vi "ProyectoInvernadero.vi"() -> ()   [LabVIEW 2020]
uses:
  <vilib>/Instr/_visa.llb/VISA Configure Serial Port (Instr).vi
  <vilib>/addons/Fuzzy Logic/FL Fuzzy Controller (SISO).vi
  <vilib>/addons/Fuzzy Logic/NI_Fuzzy_Logic_API.lvlib
panel:
  out "Error":dbl(graph)
  out "Temperatura":i32(graph)
  out "Temperatua medida":i32
  in  "Detener":bool
  out "Salida de sis Difuso":dbl
  out "String que se envia a arduino":string
  out "PWM":i32
  out "Error":dbl
  in  "Temperatura deseada":dbl
  in  "Puerto para comunicacion UART":refnum<visa-resource-name>
  in  "Archivo del Sistema Difuso":path
  # "García Nieves Alexis\nHerrera Álvarez Israel \nRamos García Abner David"
  # "Instituto Politécnico Nacional"
  # "Unidad Profesional de Ingenierias"
  # "Campus Zacatecas"
  # "Control Difuso de Temperatura para Invernadero"
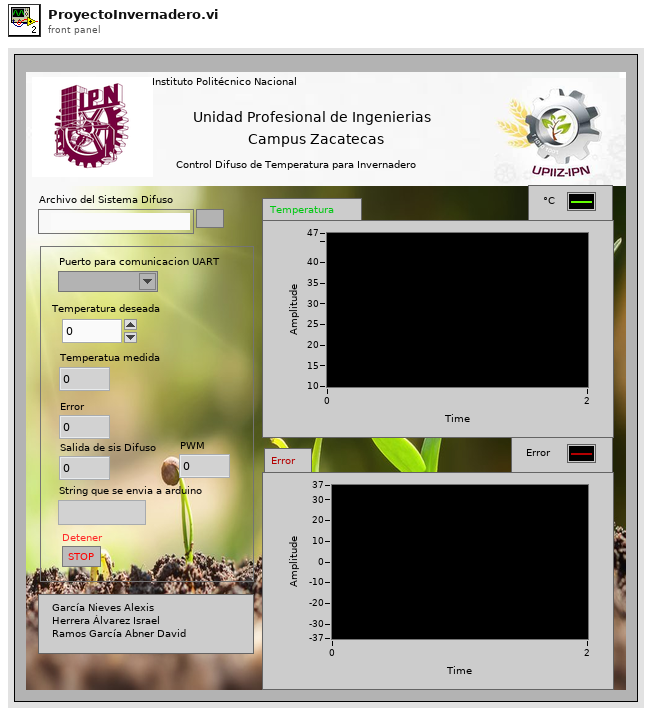
[diagram p1: front panel]
types:
  T1 = typedef "NI_Fuzzy_Logic_API.lvlib/FL System.ctl" = cluster{"input variables":T2[], "output variables":T2[], "rules":T5[], "defuzzification method":T11, "description":string, "user MF interpolating polynomials":T12[]}
  T2 = typedef "NI_Fuzzy_Logic_API.lvlib/FL Variable.ctl" = cluster{"name":string, "range":dbl[], "MFs":T3[]}
  T3 = typedef "NI_Fuzzy_Logic_API.lvlib/FL Membership Function.ctl" = cluster{"name":string, "shape":T4, "points":dbl[], "color":u32, "user-defined shape index":i32}
  T4 = typedef "NI_Fuzzy_Logic_API.lvlib/FL Membership Function Shape.ctl" = u16
  T5 = typedef "NI_Fuzzy_Logic_API.lvlib/FL Rule.ctl" = cluster{"antecedents":T6[], "antecedent connective":T8, "consequents":T9[], "consequent implication":T10, "degree of support":dbl}
  T6 = typedef "NI_Fuzzy_Logic_API.lvlib/FL Antecedent.ctl" = cluster{"Var Index":i32, "MF Index":i32, "Cond":T7}
  T7 = typedef "NI_Fuzzy_Logic_API.lvlib/FL Modifier.ctl" = u16
  T8 = typedef "NI_Fuzzy_Logic_API.lvlib/FL Antecedent Connective.ctl" = u16
  T9 = typedef "NI_Fuzzy_Logic_API.lvlib/FL Consequent.ctl" = cluster{"Var Index":i32, "MF Index":i32, "Cond":T7}
  T10 = typedef "NI_Fuzzy_Logic_API.lvlib/FL Consequent Implication.ctl" = u16
  T11 = typedef "NI_Fuzzy_Logic_API.lvlib/FL Defuzzification.ctl" = u16
  T12 = typedef "NI_Fuzzy_Logic_API.lvlib/FL Interpolating polynomials.ctl" = cluster{"X":dbl[], "Y":dbl[], "Y(x) coeff":dbl[][], "X(y) coeff":dbl[][], "Area(y) coeff":dbl[][], "coa_x(y) coeff":dbl[][]}
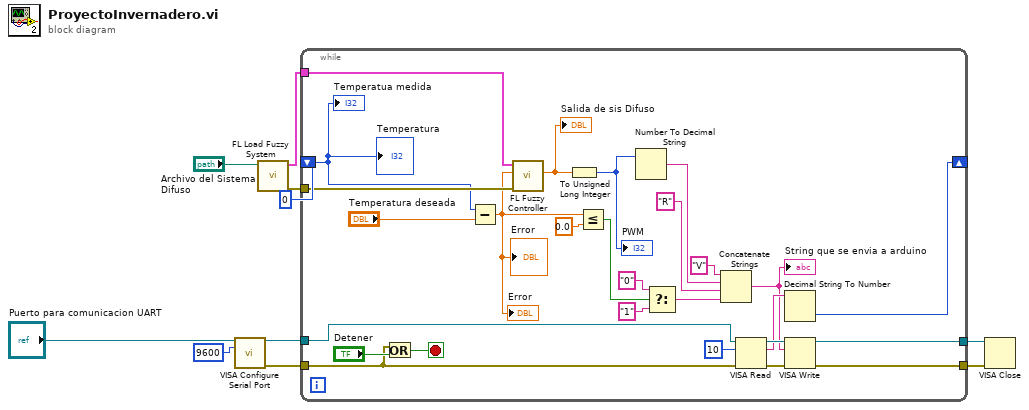
[diagram p0: block diagram]
diagram:
  n1 = call-poly "VISA Configure Serial Port"("VISA resource name"="Puerto para comunicacion UART", "baud rate (9600)"=u32 9600) -> ("VISA resource name out"=w4:refnum<visa-resource-name>, "error out"=w5:errorcluster)  [unwired: 12 in]
  n2 = call <vilib>:"FL Load Fuzzy System.vi"("file path"="Archivo del Sistema Difuso") -> ("error out"=w8:errorcluster, "fuzzy system out"=w9:T1)  [unwired: 9 in]
  n3 = while {
    tunnel: w9 -> [w37]
    tunnel: w8 -> [w36]
    tunnel: w5 -> [w18]
    tunnel: w4 -> [w17]
    shift-right: [w31] -> _
    shift-left: 0 -> [w30]
    tunnel: [w13] -> w3
    tunnel: [w12] -> w2
    stop <- w23 stop-if-true
    n4 = Or(x=w18, y="Detener") -> (x .or. y?=w23:bool)
    n5 = Subtract(x=w30, y="Temperatura deseada") -> (x-y=w20:dbl)
    "Error" <- w20
    "Error" <- w20
    n6 = call-poly <vilib>:"FL Fuzzy Controller.vi"("error in (no error)"=w36, "input value"=w20, "fuzzy system in"=w37) -> ("output value"=w32:dbl)  [unwired: 4 in, 4 out]
    "Salida de sis Difuso" <- w32
    n7 = To Unsigned Long Integer(number=w32) -> (unsigned 32bit integer=w21:u32)
    "PWM" <- w21
    n8 = Less Or Equal?(x=w20, y=0.0) -> (x <= y?=w28:bool)
    n9 = Number To Decimal String(number=w21) -> (decimal integer string=w35:string)  [unwired: 1 in]
    n10 = Select(t="0", s=w28, f="1") -> (s? t:f=w25:string)
    n11 = Concatenate Strings("V" ("string"), w35, "R" ("string"), w25) -> (w11:string)
    "String que se envia a arduino" <- w11
    n12 = VISA Read(VISA resource name=w17, byte count=u32 10, error in (no error)=w18) -> (VISA resource name out=w16:refnum<visa-resource-name>, read buffer=w14:string, error out=w15:errorcluster)  [unwired: 1 out]
    n13 = Decimal String To Number(string=w14) -> (number=w31:i32)  [unwired: 2 in, 1 out]
    n14 = VISA Write(VISA resource name=w16, write buffer=w11, error in (no error)=w15) -> (VISA resource name out=w13:refnum<visa-resource-name>, error out=w12:errorcluster)  [unwired: 1 out]
    "Temperatua medida" <- w30
    "Temperatura" <- w30
  }
  n15 = VISA Close(VISA resource name=w3, error in (no error)=w2) -> ()  [unwired: 1 out]
